vi "Format Text From Progress State.vi"(10 "Canceled":bool, 11 "Enum":T1) -> (3 "String":string)   [LabVIEW 2011]
uses:
  UI typedefs/Progress States.ctl
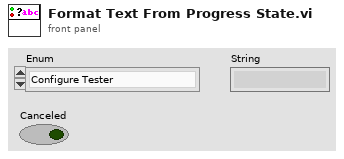
[diagram p1: front panel]
types:
  T1 = typedef "Progress States.ctl" = enum16{"Configure Tester", "Find Fiducials", "Review Fiducials", "Inspect Modules", "Review Modules", "Fill Sylgard", "Align Needle", "Purge", "Pot"}
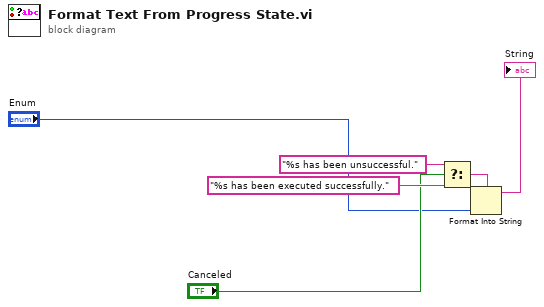
[diagram p0: block diagram]
diagram:
  n1 = Select(t="%s has been unsuccessful.", s="Canceled", f="%s has been executed successfully." ("format string")) -> (s? t:f=w5:string)
  n2 = Format Into String(format string=w5, "Enum") -> (resulting string=→"String":string)  [unwired: 2 in, 1 out]
